vi "GT_Write_Config.vi"(4 "error in (no error)":errorcluster, 7 "Config Refnum":T1) -> (0 "error out":errorcluster, 3 "refnum out":T1)   [LabVIEW 2015]
uses:
  <vilib>/Utility/config.llb/Config Data RefNum.ctl
  GSP_GT_Global.vi
  <vilib>/Utility/config.llb/Write Key (I32).vi
  <vilib>/Utility/config.llb/NI_LVConfig.lvlib
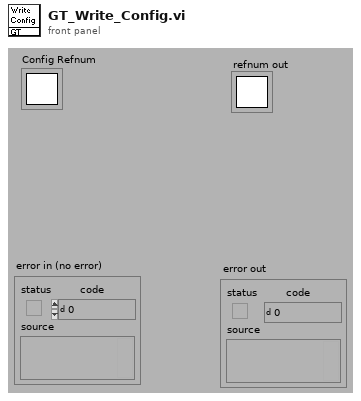
[diagram p1: front panel]
types:
  T1 = typedef "NI_LVConfig.lvlib/Config Data RefNum.ctl" = refnum<k1>
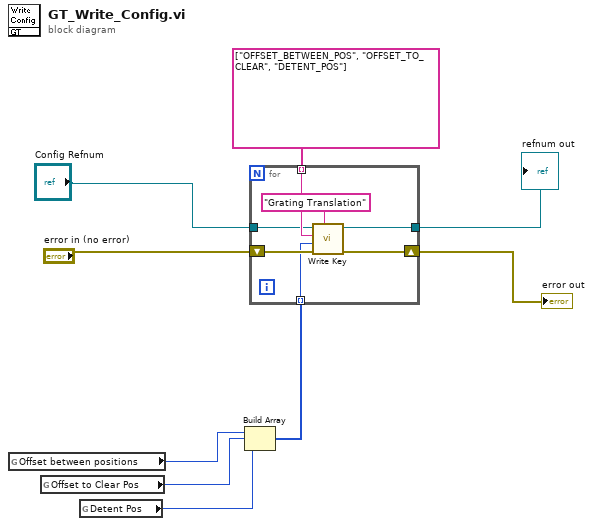
[diagram p0: block diagram]
diagram:
  n1 = global read "GSP_GT_Global.vi" "Offset between positions"() -> (w3:i32)
  n2 = global read "GSP_GT_Global.vi" "Offset to Clear Pos"() -> (w2:i32)
  n3 = global read "GSP_GT_Global.vi" "Detent Pos"() -> (w1:i32)
  n4 = Build Array(w3, w2, w1) -> (w9:i32[])
  n5 = for {
    shift-right: [w14] -> w4
    shift-left: "error in (no error)" -> [w16]
    tunnel: [w13] -> w5
    tunnel: w9 -> [w10] mode=indexing
    tunnel: string[] ["OFFSET_BETWEEN_POS", "OFFSET_TO_CLEAR", "DETENT_POS"] -> [w12] mode=indexing
    tunnel: "Config Refnum" -> [w11]
    n6 = call-poly <vilib>:"Write Key.vi"("section"="Grating Translation", "error in (no error)"=w16, "value"=w10, "key"=w12, "refnum"=w11) -> ("error out"=w14:errorcluster, "refnum out"=w13:T1)  [unwired: 4 in, 1 out]
  }
  "error out" <- w4
  "refnum out" <- w5
